vi "Recognition.Salva.vi"(8 "error in (no error)":errorcluster, 11 "Senha":string) -> (0 "error out":errorcluster)   [LabVIEW 2019]
uses:
  <vilib>/Utility/xml.llb/Write to XML File(string).vi
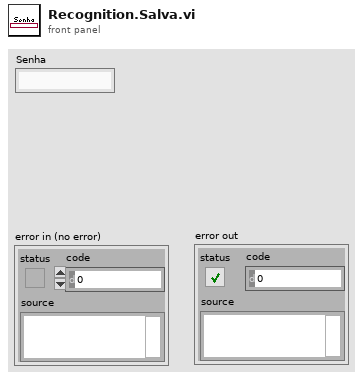
[diagram p1: front panel]
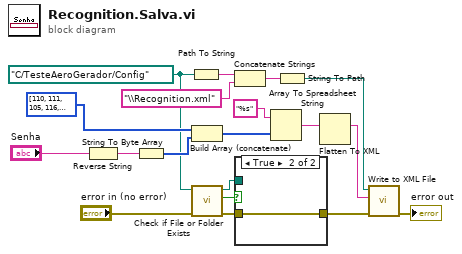
[diagram p0: block diagram]
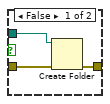
[diagram p2: hidden frame]
diagram:
  w6 = path "C:/TesteAeroGerador/Config" ("XML File Path")
  n1 = Reverse String(1:"Senha") -> (0:w9:string)
  n2 = String To Byte Array(string=w9) -> (unsigned byte array=w7:u8[])
  n3 = Path To String(path=w6) -> (string=w5:string)
  n4 = Build Array (concatenate)(u8[] [110, 111, 105, 116, 105, 110, 103, 111, 99, 101, 82] ("unsigned byte array"), w7) -> (w17:u8[])
  n5 = call <vilib>:"Check if File or Folder Exists.vi"("error in (no error)"="error in (no error)", "path"=w6) -> ("error out"=w14:errorcluster, "file or folder exists?"=w15:bool, "dup path"=w1:path)  [unwired: 7 in]
  n6 = Concatenate Strings(w5, "\\Recognition.xml") -> (w3:string)
  n7 = case shown="True" w15 {
    tunnel: w1 -> [w22 _]
    tunnel: w14 -> [w21 w23]
    tunnel: [w20 w23] -> w12
    frame False {
      n8 = Create Folder(path (use dialog)=w22, error in=w21) -> (error out=w20:errorcluster)  [unwired: 1 in, 2 out]
    }
    frame True {
    }
  }
  n9 = Array To Spreadsheet String(array=w17, 3:"%s" ("format string")) -> (spreadsheet string=w16:string)  [unwired: 1 in]
  n10 = String To Path(string=w3) -> (path=w2:path)
  n11 = Flatten To XML(anything=w16) -> (xml string=w11:string)
  n12 = call-poly <vilib>:"Write to XML File.vi"("error in (no error)"=w12, "XML Input"=w11, "XML File Path"=w2) -> ("error out"=→"error out":errorcluster)  [unwired: 6 in, 2 out]
